vi "Initialize.vi"(8 "error in":errorcluster, 11 "Plugin in":refnum<class "Spectrogram.lvclass">) -> (0 "error out":errorcluster, 3 "Plugin out":refnum<class "Spectrogram.lvclass">)   [LabVIEW 2023, in "Spectrogram.lvlib" / "Spectrogram.lvclass"]
uses:
  Spectrogram.lvclass
  C:/Program Files/National Instruments/LabVIEW 2023/vi.lib/FlexLogger/SDK/PluginSDK.lvlibp/PEFClasses/SDK/Plugin/Plugin.lvclass
  Spectrogram Global.vi
  <vilib>/FlexLogger/SDK/PluginSDK.lvlibp/PEFClasses/SDK/Plugin/ParameterAccess/Write Single Channel.vi
  <vilib>/FlexLogger/SDK/PluginSDK.lvlibp/PEFClasses/SDK/Plugin/ParameterAccess/Write Enum.vi
  <vilib>/FlexLogger/SDK/PluginSDK.lvlibp/PEFClasses/SDK/Plugin/ParameterAccess/Write I32.vi
  <vilib>/FlexLogger/SDK/PluginSDK.lvlibp/PEFClasses/SDK/Plugin/ParameterAccess/Write Command.vi
  <vilib>/FlexLogger/SDK/PluginSDK.lvlibp/PEFClasses/SDK/Plugin/Plugin.lvclass
  C:/Program Files/National Instruments/LabVIEW 2023/vi.lib/FlexLogger/SDK/PluginSDK.lvlibp/PEFClasses/SDK/Processing Element/Processing Element.lvclass
  C:/Users/Localization Tester/Documents/LabVIEW Projects/FlexLogger IO Plug-ins/Spectrogram/Spectrogram.lvclass
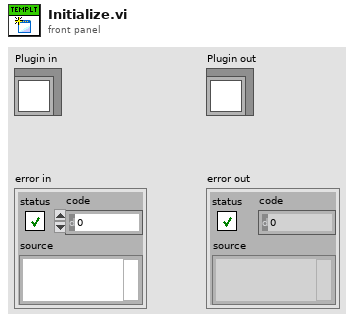
[diagram p1: front panel]
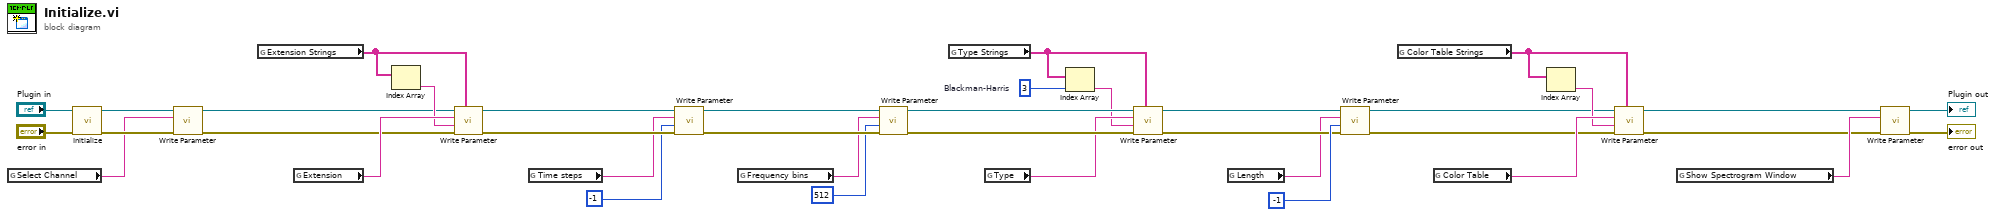
[diagram p0: block diagram]
diagram:
  w13 = 3  # Blackman-Harris
  n1 = global read "Spectrogram Global.vi" "Select Channel"() -> (w21:string)
  n2 = call-parent "Initialize.vi"("error in (no error)"="error in", "Plugin in"="Plugin in") -> ("error out"=w35:errorcluster, "Plugin out"=w36:refnum<class "Spectrogram.lvclass">)  [unwired: 8 in]
  n3 = call-poly <vilib>:"Write Parameter.vi"("error in (no error)"=w35, "Name (Unique Channel Identifier)"=w21, "Plugin in"=w36) -> ("error out"=w1:errorcluster, "Plugin out"=w2:refnum<class "Spectrogram.lvclass">)  [unwired: 7 in]
  n4 = global read "Spectrogram Global.vi" "Extension Strings"() -> (w19:string[])
  n5 = global read "Spectrogram Global.vi" "Extension"() -> (w20:string)
  n6 = Index Array(array=w19) -> (element=w18:string)  [unwired: 1 in]
  n7 = call-poly <vilib>:"Write Parameter.vi"("Possible Values"=w19, "error in (no error)"=w1, "Current Value"=w18, "Name"=w20, "Plugin in"=w2) -> ("error out"=w33:errorcluster, "Plugin out"=w34:refnum<class "Spectrogram.lvclass">)  [unwired: 5 in]
  n8 = global read "Spectrogram Global.vi" "Time steps"() -> (w17:string)
  n9 = call-poly <vilib>:"Write Parameter.vi"("error in (no error)"=w33, "Value"=-1, "Name"=w17, "Plugin in"=w34) -> ("error out"=w30:errorcluster, "Plugin out"=w31:refnum<class "Spectrogram.lvclass">)  [unwired: 6 in]
  n10 = global read "Spectrogram Global.vi" "Frequency bins"() -> (w16:string)
  n11 = call-poly <vilib>:"Write Parameter.vi"("error in (no error)"=w30, "Value"=512, "Name"=w16, "Plugin in"=w31) -> ("error out"=w27:errorcluster, "Plugin out"=w28:refnum<class "Spectrogram.lvclass">)  [unwired: 6 in]
  n12 = global read "Spectrogram Global.vi" "Type Strings"() -> (w14:string[])
  n13 = global read "Spectrogram Global.vi" "Type"() -> (w15:string)
  n14 = Index Array(array=w14, index=w13) -> (element=w12:string)
  n15 = call-poly <vilib>:"Write Parameter.vi"("Possible Values"=w14, "error in (no error)"=w27, "Current Value"=w12, "Name"=w15, "Plugin in"=w28) -> ("error out"=w24:errorcluster, "Plugin out"=w26:refnum<class "Spectrogram.lvclass">)  [unwired: 5 in]
  n16 = global read "Spectrogram Global.vi" "Length"() -> (w11:string)
  n17 = call-poly <vilib>:"Write Parameter.vi"("error in (no error)"=w24, "Value"=-1, "Name"=w11, "Plugin in"=w26) -> ("error out"=w4:errorcluster, "Plugin out"=w6:refnum<class "Spectrogram.lvclass">)  [unwired: 6 in]
  n18 = global read "Spectrogram Global.vi" "Color Table Strings"() -> (w8:string[])
  n19 = global read "Spectrogram Global.vi" "Color Table"() -> (w9:string)
  n20 = Index Array(array=w8) -> (element=w7:string)  [unwired: 1 in]
  n21 = call-poly <vilib>:"Write Parameter.vi"("Possible Values"=w8, "error in (no error)"=w4, "Current Value"=w7, "Name"=w9, "Plugin in"=w6) -> ("error out"=w3:errorcluster, "Plugin out"=w5:refnum<class "Spectrogram.lvclass">)  [unwired: 5 in]
  n22 = global read "Spectrogram Global.vi" "Show Spectrogram Window"() -> (w10:string)
  n23 = call-poly <vilib>:"Write Parameter.vi"("error in (no error)"=w3, "Name"=w10, "Plugin in"=w5) -> ("error out"=→"error out":errorcluster, "Plugin out"=→"Plugin out":refnum<class "Spectrogram.lvclass">)  [unwired: 7 in]
